vi "Global_ACT_Data Out.vi"() -> ()   [LabVIEW 2020, in "Sholder_ACT.lvlib"]
uses:
  startup.rtexe/Sholder_ACT.lvlib
  startup.rtexe/CTRE_Phoenix_MotorControl_ControlMode.ctl
  startup.rtexe/Cluster_Sholder_HW Outputs.ctl
  startup.rtexe/Cluster_FX Sensor Values.ctl
  startup.rtexe/Cluster_FX CloseLoop Values.ctl
  startup.rtexe/Cluster_FX Limit Switchs.ctl
  startup.rtexe/Cluster_FX Current Values.ctl
  startup.rtexe/Cluster_FX Integrated Sensor Values.ctl
  startup.rtexe/Cluster_Sholder_SW Output Data.ctl
panel:
  in  "ACT_Sholder_SW Outputs":T1
  out "ACT_Sholder_HW Outputs":T2
  in  "ACT_Sholder_FX Mode":T8 items=["PercentOutput"=0, "Position"=1, "Velocity"=2, "Current"=3, "Follower"=5, "MotionProfile"=6, "MotionMagic"=7, "MotionProfileArc"=10, "Disabled"=15]
  in  "ACT_Sholder_FX Value":dbl
  in  "ACT_Sholder_CycleTime(S)":dbl
  # "The Names of the Data items in the Global Variable MUST describe who the Single Writer is\nFor Actuator Globals the the naming convention is\n   \nACT_Lib Name_Data Name\n\nExamples:\nACT_Drive_X axis\nACT_Hopper_AgitatorSpeed"
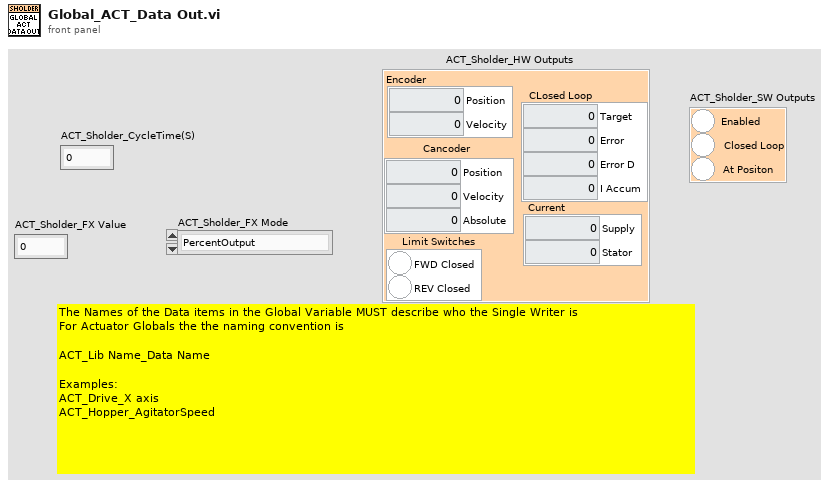
[diagram p1: front panel]
types:
  T1 = typedef "Cluster_Sholder_SW Output Data.ctl" = cluster{"Enabled":bool, "Closed Loop":bool, "At Positon":bool}
  T2 = typedef "Cluster_Sholder_HW Outputs.ctl" = cluster{"Encoder":T3, "CLosed Loop":T4, "Limit Switches":T5, "Current":T6, "Cancoder":T7}
  T3 = typedef "Cluster_FX Sensor Values.ctl" = cluster{"Position":i32, "Velocity":i32}
  T4 = typedef "Cluster_FX CloseLoop Values.ctl" = cluster{"Target":dbl, "Error":i32, "Error D":dbl, "I Accum":dbl}
  T5 = typedef "Cluster_FX Limit Switchs.ctl" = cluster{"FWD Closed":bool, "REV Closed":bool}
  T6 = typedef "Cluster_FX Current Values.ctl" = cluster{"Supply":dbl, "Stator":dbl}
  T7 = typedef "Cluster_FX Integrated Sensor Values.ctl" = cluster{"Position":dbl, "Velocity":dbl, "Absolute":dbl}
  T8 = typedef "CTRE_Phoenix_MotorControl_ControlMode.ctl" = u16
diagram:
